vi "Main.vi"() -> ()   [LabVIEW 2020]
uses:
  Def/Queue_Function Def.ctl
  Def/Queue_Method Def.ctl
  Def/Error handler.ctl
  Def/MHL_Data.ctl
  Def/User_Event.ctl
  Main Support/Main Sub Vi/Def/Module names.ctl
  Def/Queue_Def.ctl
  Main Support/Error Handling/Error Handler.lvlib
  DQMH Modules/Module.lvlib
  <vilib>/Utility/Data Type/NI_Data Type.lvlib
panel:
  out "Ver.#":string
  out "error out":errorcluster
  in  "error in (no error)":errorcluster
  # "客戶購買記帳「」\n    顯示客戶清單\n    按下「客戶清單」顯示該客戶上次採買項目\n    按下「品項紀錄」顯示該客戶買過哪些產品、價格\n    按下「新增客戶」可在「客戶清單」顯示新增\n吐出月報表\n    1. 匯出該月、該季、半年、全年營業額\n    2. 匯出個客戶該月、該季、半年、全年營業額\n\n該客戶超過該週期未購買警報\n--->自動掃描模式"
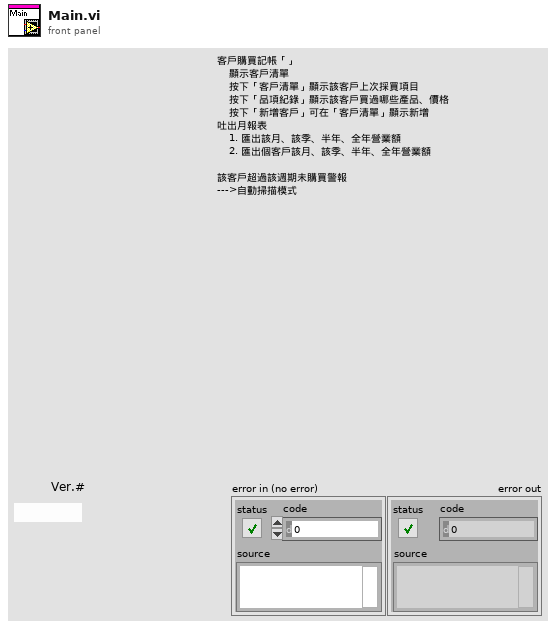
[diagram p1: front panel]
types:
  T1 = typedef "User_Event.ctl" = cluster{"String":string, "Data":variant}
  T2 = enum16{"Initialize", "Get", "Read", "Write", "Release"}
  T3 = typedef "MHL_Data.ctl" = cluster{"String":string}
  T4 = typedef "Error handler.ctl" = cluster{"code":i32, "source":string}
  T5 = typedef "Queue_Method Def.ctl" = enum16{"Initialize", "Read", "Write", "Insert", "Get_Specific_Quene_Status", "Flush Speciffic Quene", "Release All Quenes"}
  T6 = typedef "Queue_Function Def.ctl" = enum16{"MHL", "Return(Watch dog)", "Event Log", "Error Log"}
  T7 = typedef "Main_Data_Package.ctl" = cluster{"This Vi Ref Out":refnum<vi>, "Map Out":map{string, refnum<vi>}, "User Event Ref":refnum<user-event>, "Event Log Path":path}
  T8 = typedef "Module.lvlib/Broadcast Events--cluster.ctl" = cluster{"Module Did Init":refnum<user-event>, "Status Updated":refnum<user-event>, "Error Reported":refnum<user-event>, "Module Did Stop":refnum<user-event>, "Update Module Execution Status":refnum<user-event>}
  T9 = cluster{"Functions":T6, "Functions 2":T6, "Functions 3":T6, "Functions 4":T6}
  T10 = typedef "Queue_Def.ctl" = cluster{"Message":string, "Data":variant}
  T11 = typedef "Module names.ctl" = enum16{"Module"}
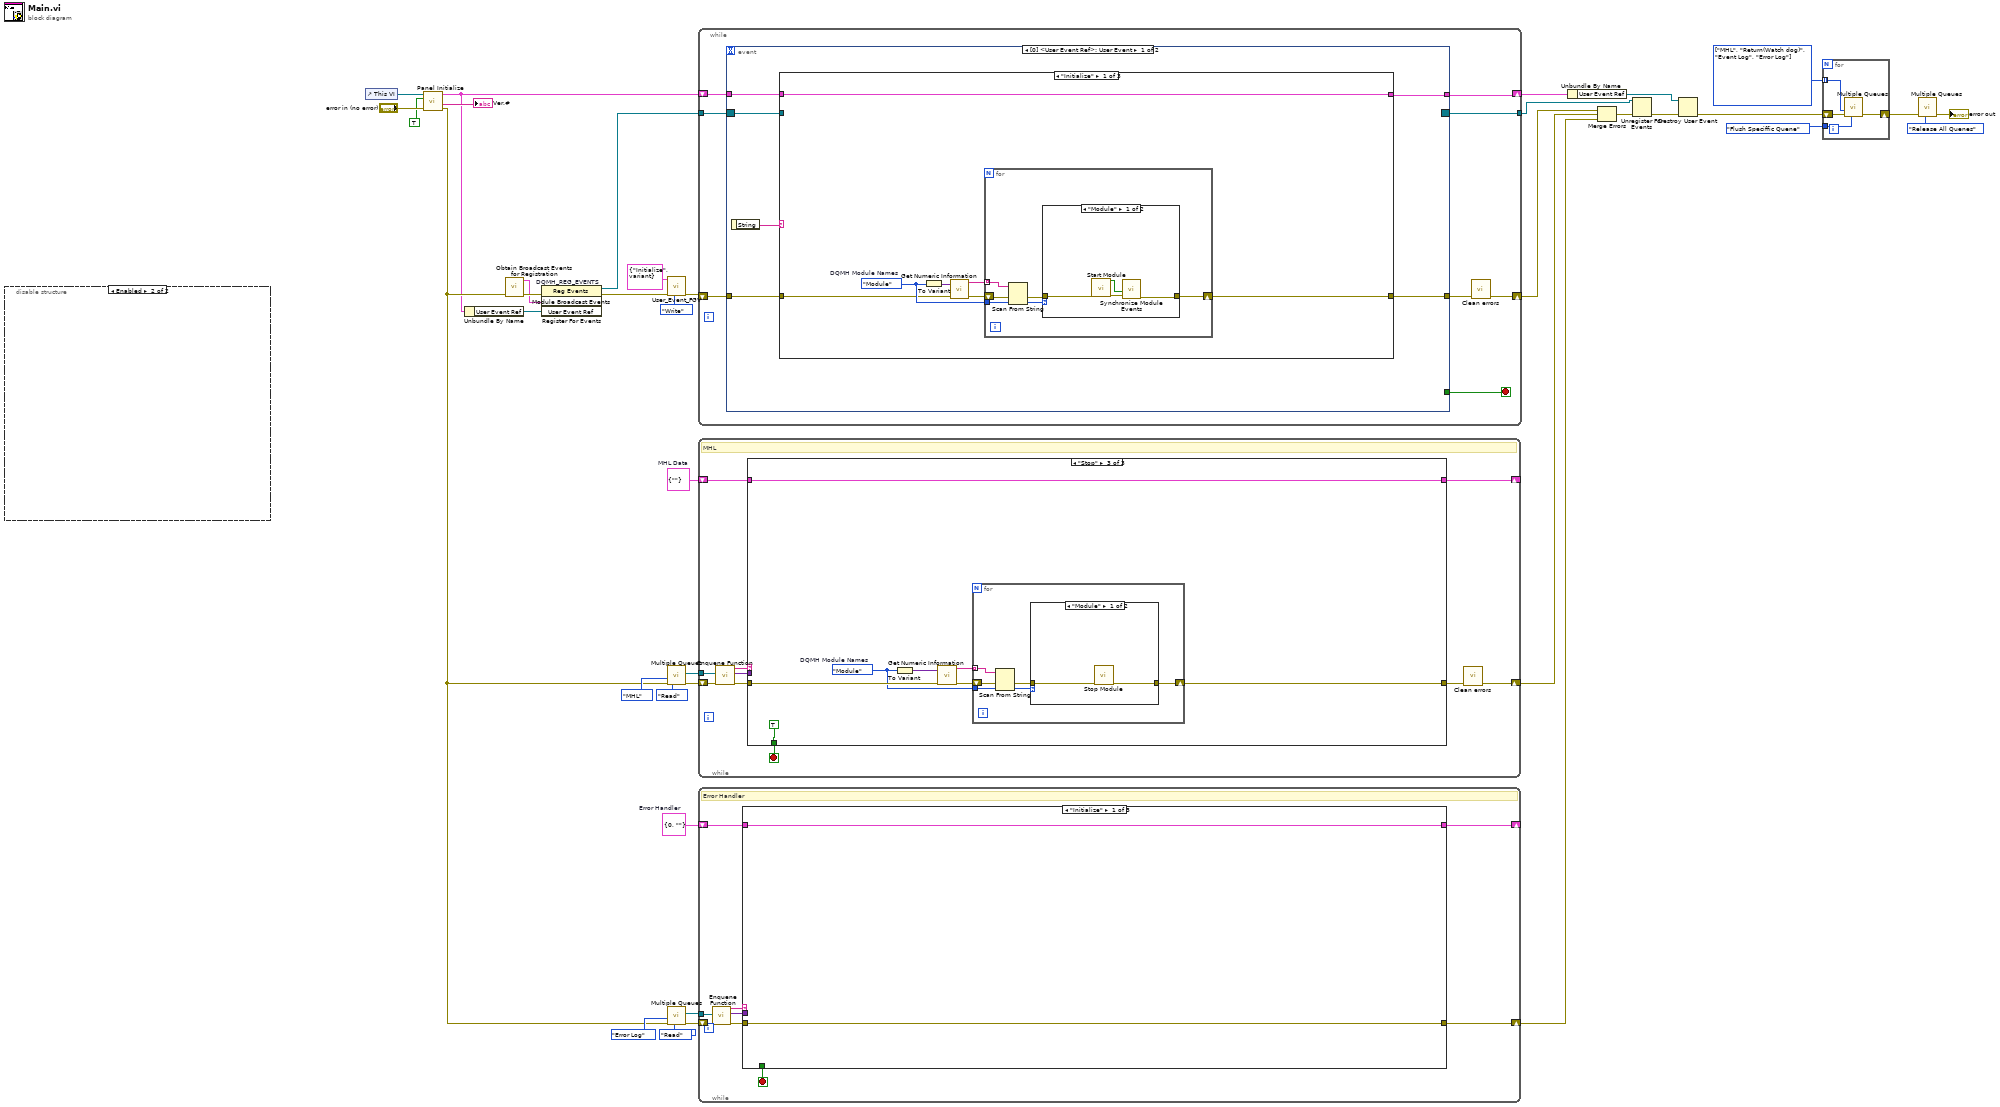
[diagram p0: block diagram]
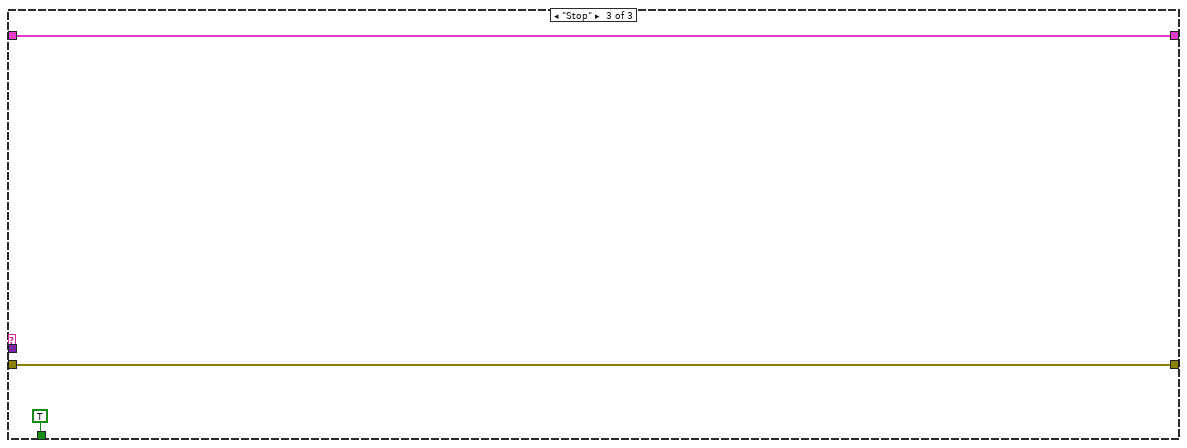
[diagram p4: hidden frame]
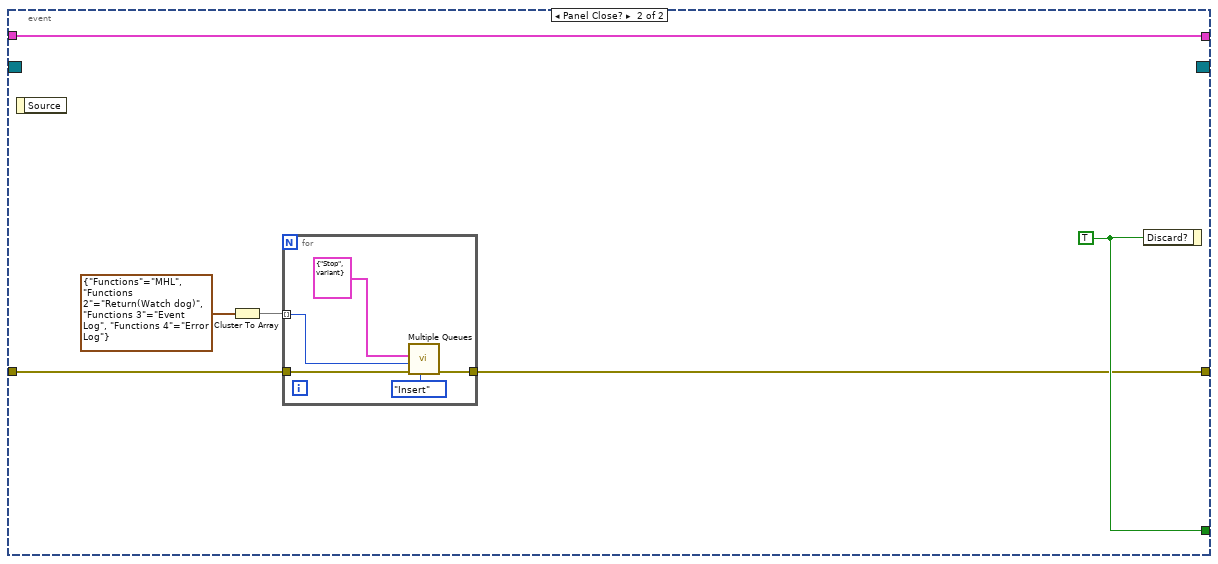
[diagram p11: hidden frame]
diagram:
  w24 = T3 {"String"=""}  # MHL Data
  w13 = T4 {"code"=0, "source"=""}  # Error Handler
  w32 = T6[] [enum."MHL", enum."Return(Watch dog)", enum."Event Log", enum."Error Log"] items=["MHL", "Return(Watch dog)", "Event Log", "Error Log"]
  n1 = disable-structure shown="Enabled" {
    frame Disabled {
    }
    frame Enabled {
    }
  }
  n2 = control-ref of="This VI"() -> (w38:refnum<vi>)
  n3 = call "Panel Initialize.vi"("error in"="error in (no error)", "Initialize All UI ?"=TRUE, "VI Ref"=w38) -> ("error out"=w6:errorcluster, "Ver.#"=→"Ver.#":string, "Structure Data"=w5:T7)  [unwired: 6 in]
  n4 = Unbundle By Name(w5) -> ("User Event Ref"=w2:refnum<user-event>)
  n5 = call "Obtain Broadcast Events for Registration.vi"("error in"=w6) -> ("error out"=w4:errorcluster, "Module Broadcast Events"=w3:T8)  [unwired: 8 in, 1 out]
  n6 = register-events "DQMH_REG_EVENTS"(error in=w4, w3, w2) -> (reference out=w1:refnum<event-registration>, error out=w10:errorcluster)  [unwired: 1 in]
  n7 = call "User_Event_FGV.vi"("Method"=T2."Write", "error in"=w10, "User Event"=T1 {"String"="Initialize", "Data"=variant}) -> ("error out"=w7:errorcluster)  [unwired: 7 in, 1 out]
  n8 = call "Multiple Queues.vi"("Method"=Queue_Method_Def."Read", "error in"=w6, "Functions"=Queue_Function_Def."MHL") -> ("error out"=w20:errorcluster, "queue out"=w21:refnum<queue>)  [unwired: 6 in, 1 out]
  n9 = call "Multiple Queues.vi"("Method"=Queue_Method_Def."Read", "error in"=w6, "Functions"=Queue_Function_Def."Error Log") -> ("error out"=w15:errorcluster, "queue out"=w14:refnum<queue>)  [unwired: 6 in, 1 out]
  n10 = while {
    tunnel: [w45] -> w11
    shift-right: [w40] -> w35
    shift-left: w7 -> [w44]
    shift-right: [w42] -> w19
    shift-left: w5 -> [w43]
    tunnel: w1 -> [w39]
    stop <- w46 stop-if-true
    n11 = event shown="[0] <User Event Ref>: User Event" {
      selector: w39 -> [w47 _]
      dyn-events: [_ _] -> w45
      timeout: _ -> [_ _]
      tunnel: [_ w80] -> w46
      tunnel: w44 -> [w52 w79]
      tunnel: [w51 w75] -> w41
      tunnel: w43 -> [w49 w76]
      tunnel: [w48 w76] -> w42
      event User Event {
        n12 = event-data() -> ("String"=w50:string)  [unwired: 1 in]
        n13 = case shown="\"Initialize\"" w50 {
          tunnel: w52 -> [w54 w72 w74]
          tunnel: [w53 w72 w74] -> w51
          tunnel: [w59 w71 w73] -> w48
          tunnel: w49 -> [w59 w71 w73]
          tunnel: w47 -> [_ _ _]
          frame "Initialize" {
            w55 = Module_names."Module"  # DQMH Module Names
            n14 = To Variant(anything=w55) -> (Variant=w58:variant)
            n15 = call <vilib>:"Get Numeric Information.vi"("error in (no error)"=w54, "variant"=w58) -> ("error out"=w57:errorcluster, "enum names"=w56:string[])  [unwired: 6 in, 2 out]
            n16 = for {
              shift-right: [w65] -> w53
              shift-left: w57 -> [w64]
              tunnel: w56 -> [w60] mode=indexing
              tunnel: w55 -> [w62]
              n17 = Scan From String(input string=w60, error in=w64, default 1=w62) -> (error out=w63:errorcluster, output 1=w61:T11)  [unwired: 2 in, 2 out]
              n18 = case shown="\"Module\"" w61 {
                tunnel: w63 -> [w67 w70]
                tunnel: [w66 w70] -> w65
                frame "Module" {
                  n19 = call "Start Module.vi"("error in"=w67) -> ("error out"=w68:errorcluster, "Module Was Already Running?"=w69:bool)  [unwired: 7 in, 2 out]
                  n20 = call "Synchronize Module Events.vi"("error in"=w68, "Wait for Event Sync?"=w69) -> ("error out"=w66:errorcluster)  [unwired: 9 in]
                }
                frame Default {
                }
              }
            }
          }
          frame "Refresh" {
          }
          frame Default {
          }
        }
      }
      event Panel Close? {
        w80 = TRUE ("Discard?")
        n21 = event-data() -> ()  [unwired: 1 in, 1 out]
        n22 = Cluster To Array(cluster=T9 {"Functions"=enum."MHL", "Functions 2"=enum."Return(Watch dog)", "Functions 3"=enum."Event Log", "Functions 4"=enum."Error Log"}) -> (array=w77:T6[])
        n23 = for {
          tunnel: w77 -> [w82] mode=indexing
          tunnel: w79 -> [w85]
          tunnel: [w84] -> w75
          n24 = call "Multiple Queues.vi"("Method"=Queue_Method_Def."Insert", "error in"=w85, "Functions"=w82, "Quenes"=T10 {"Message"="Stop", "Data"=variant}) -> ("error out"=w84:errorcluster)  [unwired: 5 in, 2 out]
        }
        n25 = event-data("Discard?"=w80) -> ()  [unwired: 1 in, 1 out]
      }
    }
    n26 = call "Clean errors.vi"("error in (no error)"=w41) -> ("error out"=w40:errorcluster)  [unwired: 10 in]
  }
  n27 = while {
    shift-right: [w86] -> w34
    shift-left: w20 -> [w88]
    shift-right: [w90] -> _
    shift-left: w24 -> [w87]
    tunnel: w21 -> [w89]
    stop <- w95 stop-if-true
    # "MHL"
    n28 = call "Enquene Function.vi"("error in (no error)"=w88, "Queue"=w89) -> ("error out"=w93:errorcluster, "Data"=w91:variant, "Message"=w92:string)  [unwired: 7 in]
    n29 = case shown="\"Stop\"" w92 {
      tunnel: [_ _ TRUE] -> w95
      tunnel: [w97 w99 w105] -> w94
      tunnel: w93 -> [w97 w99 w103]
      tunnel: w91 -> [_ _ _]
      tunnel: [w96 w98 w106] -> w90
      tunnel: w87 -> [w96 w98 w106]
      frame "Initialize" {
      }
      frame Default {
      }
      frame "Stop" {
        w100 = Module_names."Module"  # DQMH Module Names
        n30 = To Variant(anything=w100) -> (Variant=w104:variant)
        n31 = call <vilib>:"Get Numeric Information.vi"("error in (no error)"=w103, "variant"=w104) -> ("error out"=w102:errorcluster, "enum names"=w101:string[])  [unwired: 6 in, 2 out]
        n32 = for {
          shift-right: [w113] -> w105
          shift-left: w102 -> [w112]
          tunnel: w101 -> [w108] mode=indexing
          tunnel: w100 -> [w110]
          n33 = Scan From String(input string=w108, error in=w112, default 1=w110) -> (error out=w111:errorcluster, output 1=w109:T11)  [unwired: 2 in, 2 out]
          n34 = case shown="\"Module\"" w109 {
            tunnel: w111 -> [w115 w116]
            tunnel: [w114 w116] -> w113
            frame "Module" {
              n35 = call "Stop Module.vi"("error in"=w115) -> ("error out"=w114:errorcluster)  [unwired: 10 in]
            }
            frame Default {
            }
          }
        }
      }
    }
    n36 = call "Clean errors.vi"("error in (no error)"=w94) -> ("error out"=w86:errorcluster)  [unwired: 10 in]
  }
  n37 = while {
    shift-right: [w123] -> w12
    shift-left: w15 -> [w125]
    tunnel: w14 -> [w119]
    shift-right: [w117] -> _
    shift-left: w13 -> [w118]
    stop <- w120 stop-if-true
    # "Error Handler"
    n38 = call "Enquene Function.vi"("error in (no error)"=w125, "Queue"=w119) -> ("error out"=w124:errorcluster, "Data"=w121:variant, "Message"=w122:string)  [unwired: 7 in]
    n39 = case shown="\"Initialize\"" w122 {
      tunnel: [w127 w129 w131] -> w123
      tunnel: w124 -> [w127 w129 w131]
      tunnel: w121 -> [_ _ _]
      tunnel: [_ _ TRUE] -> w120
      tunnel: w118 -> [w126 w128 w130]
      tunnel: [w126 w128 w130] -> w117
      frame "Initialize" {
      }
      frame Default {
      }
      frame "Stop" {
      }
    }
  }
  n40 = Unbundle By Name(w19) -> ("User Event Ref"=w18:refnum<user-event>)
  n41 = Merge Errors(w35, w34, w12) -> (w33:errorcluster)
  n42 = Unregister For Events(event registration refnum=w11, error in=w33) -> (error out=w36:errorcluster)
  n43 = Destroy User Event(user event=w18, error in=w36) -> (error out=w31:errorcluster)
  n44 = for {
    tunnel: w32 -> [w136] mode=indexing
    shift-right: [w134] -> w30
    shift-left: w31 -> [w135]
    tunnel: Queue_Method_Def."Flush Speciffic Quene" ("Method") -> [w133]
    n45 = call "Multiple Queues.vi"("Method"=w133, "error in"=w135, "Functions"=w136) -> ("error out"=w134:errorcluster)  [unwired: 6 in, 2 out]
  }
  n46 = call "Multiple Queues.vi"("Method"=Queue_Method_Def."Release All Quenes", "error in"=w30) -> ("error out"=→"error out":errorcluster)  [unwired: 7 in, 2 out]
